vi "Remove Rows with Zeros.vi"(1 "Comparison # (default 0)":i32, 2 "Index of 0":i32, 3 "Input Array":dbl[][](array[numeric])) -> (0 "Rows with Zeros Removed":dbl[][](array[numeric]))   [LabVIEW 2011]
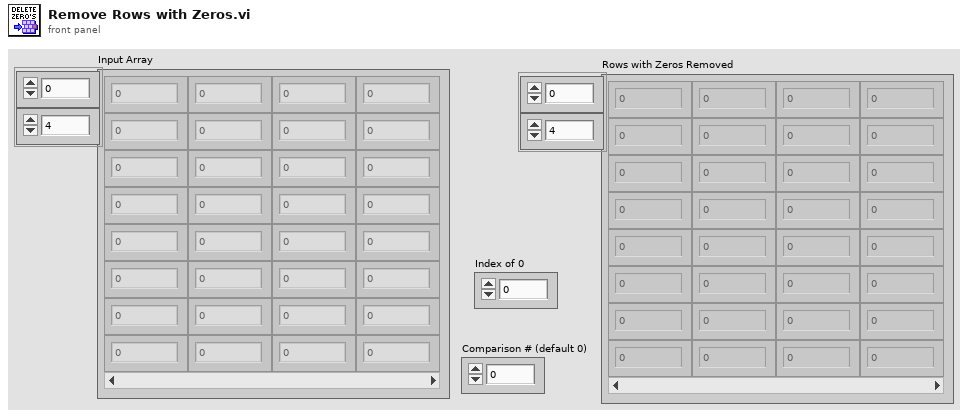
[diagram p1: front panel]
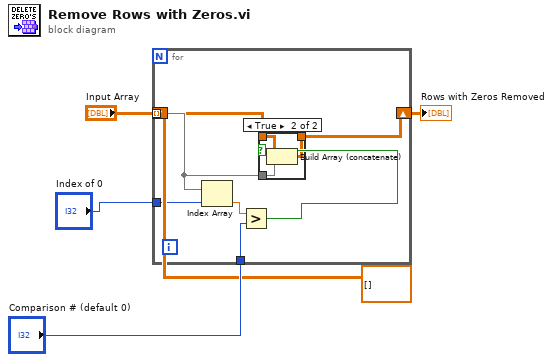
[diagram p0: block diagram]
diagram:
  n1 = for {
    tunnel: "Input Array" -> [w12] mode=indexing
    tunnel: "Index of 0" -> [w11]
    tunnel: "Comparison # (default 0)" -> [w8]
    shift-right: [w6] -> w4
    shift-left: dbl[][] [] ("Input Array 2") -> [w7]
    n2 = Index Array(array=w12, index=w11) -> (element=w9:dbl)
    n3 = Greater?(x=w9, y=w8) -> (0:w10:bool)
    n4 = case shown="True" w10 {
      tunnel: w7 -> [w13 w15]
      tunnel: w12 -> [_ w14]
      tunnel: [w13 w16] -> w6
      frame False {
      }
      frame True {
        n5 = Build Array (concatenate)(w15, w14) -> (w16:dbl[][])
      }
    }
  }
  "Rows with Zeros Removed" <- w4
